vi "DrawCursor.vi"(6 "Visible?":bool, 8 "error in (no error)":errorcluster, 10 "GameIn":refnum<class "Game.lvclass">, 11 "Highscore in":refnum<class "HighscoreDialog.lvclass">) -> (0 "error out":errorcluster, 2 "GameOut":refnum<class "Game.lvclass">, 3 "Highscore out":refnum<class "HighscoreDialog.lvclass">)   [LabVIEW 2019, in "RT_Game.lvlib" / "HighscoreDialog.lvclass"]
uses:
  HighscoreDialog/HighscoreDialog.lvclass
  C:/Users/FreshBob/Dropbox/VIs/myRIO_GameConsole/RT/RT_Game/GameObject/GameObject.lvclass
  Game/Game.lvclass
  Game/Coordinate.ctl
  GameObject/GameObject.lvclass/GameObject.ctl
  HighscoreDialog/HighscoreDialog.lvclass/HighscoreDialog.ctl
  GameObject/Read position.vi
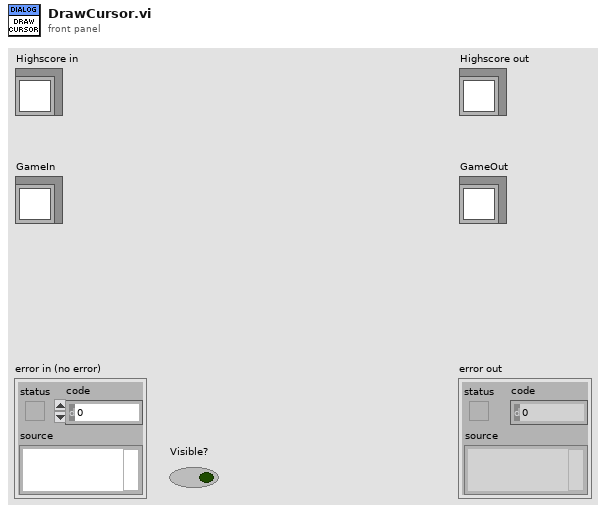
[diagram p1: front panel]
types:
  T1 = typedef "RT_Game.lvlib/Game.lvclass/Coordinate.ctl" = cluster{"x":dbl, "y":dbl}
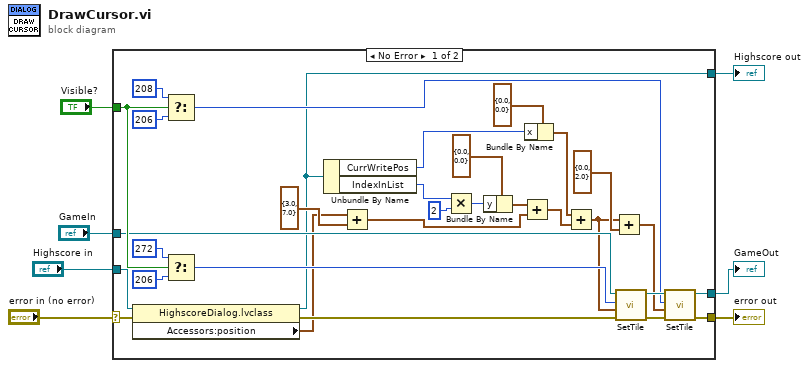
[diagram p0: block diagram]
diagram:
  n1 = case shown="No Error" "error in (no error)" {
    selector: "error in (no error)" -> [w38 w41]
    tunnel: [w36 w41] -> w6
    tunnel: [w10 w40] -> w4
    tunnel: "Highscore in" -> [w11 w40]
    tunnel: [w34 w39] -> w3
    tunnel: "GameIn" -> [w15 w39]
    tunnel: "Visible?" -> [w27 _]
    frame No Error {
      n2 = property class="HighscoreDialog.lvclass"(reference=w11, error in=w38) -> (reference out=w10:refnum<class "HighscoreDialog.lvclass">, error out=w12:errorcluster, "Accessors:position"=w9:T1)
      n3 = Select(t=u32 208 ("TileNumber"), s=w27, f=u32 206) -> (s? t:f=w28:u32)
      n4 = Select(t=u32 272 ("TileNumber"), s=w27, f=u32 206) -> (s? t:f=w32:u32)
      n5 = Unbundle By Name(w10) -> ("CurrWritePos"=w16:i16, "IndexInList"=w8:i16)
      n6 = Add(x=w9, y=T1 {"x"=3.0, "y"=7.0}) -> (x+y=w24:T1)
      n7 = Multiply(x=w8, y=i16 2) -> (x*y=w21:i16)
      n8 = Bundle By Name(cluster=T1 {"x"=0.0, "y"=0.0} ("x"), "y"=w21) -> (w22:T1)
      n9 = Add(x=w22, y=w24) -> (x+y=w13:T1)
      n10 = Bundle By Name(cluster=T1 {"x"=0.0, "y"=0.0} ("x"), "x"=w16) -> (w17:T1)
      n11 = Add(x=w17, y=w13) -> (x+y=w14:T1)
      n12 = Add(x=w14, y=T1 {"x"=0.0, "y"=2.0}) -> (x+y=w19:T1)
      n13 = call "SetTile.vi"("error in (no error)"=w12, "Coordinates"=w14, "TileNumber"=w32, "Game in"=w15) -> ("error out"=w37:errorcluster, "Game out"=w35:refnum<class "Game.lvclass">)  [unwired: 6 in]
      n14 = call "SetTile.vi"("error in (no error)"=w37, "Coordinates"=w19, "TileNumber"=w28, "Game in"=w35) -> ("error out"=w36:errorcluster, "Game out"=w34:refnum<class "Game.lvclass">)  [unwired: 6 in]
    }
    frame Error {
    }
  }
  "error out" <- w6
  "Highscore out" <- w4
  "GameOut" <- w3
